vi "Program_Run.vi"(8 "error in (no error)":errorcluster, 10 "Numeric":u16, 11 "SpinCoater in":refnum<class "SpinCoater.lvclass">) -> (0 "error out":errorcluster, 3 "SpinCoater out":refnum<class "SpinCoater.lvclass">)   [LabVIEW 2020, in "SpinCoater.lvclass"]
uses:
  <instrlib>/Classes/SpinCoater/SpinCoater.lvclass
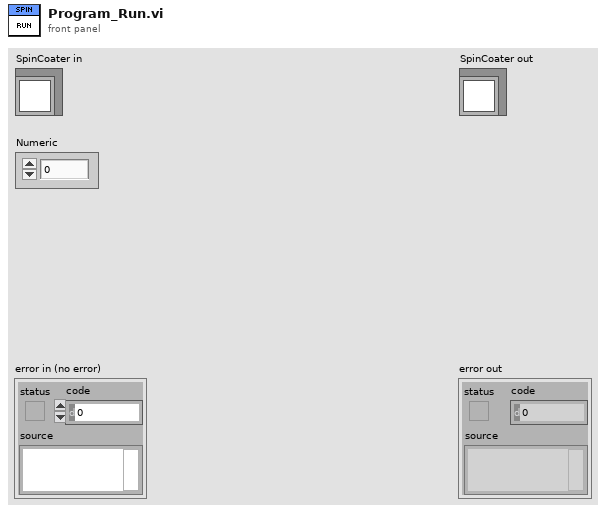
[diagram p1: front panel]
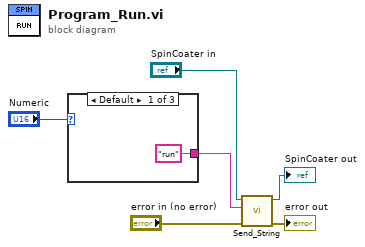
[diagram p0: block diagram]
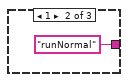
[diagram p2: hidden frame]
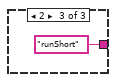
[diagram p3: hidden frame]
diagram:
  n1 = case shown="Default" "Numeric" {
    tunnel: ["run" ("write buffer") "runNormal" ("write buffer") "runShort" ("write buffer")] -> w1
    frame Default {
    }
    frame 1 {
    }
    frame 2 {
    }
  }
  n2 = call-dynamic "Send_String.vi"("error in (no error)"="error in (no error)", "String"=w1, "SpinCoater in"="SpinCoater in") -> ("error out"=→"error out":errorcluster, "SpinCoater out"=→"SpinCoater out":refnum<class "SpinCoater.lvclass">)  [unwired: 6 in, 1 out]
